vi "calculateRoll.vi"(9 "az":dbl, 10 "ay":dbl) -> (3 "roll":dbl)   [LabVIEW 2019]
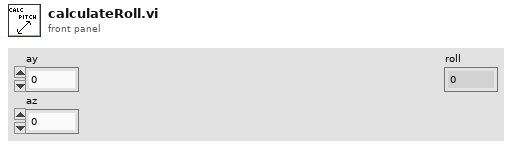
[diagram p1: front panel]
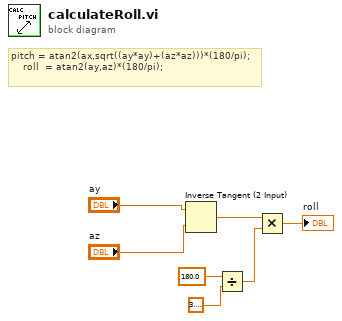
[diagram p0: block diagram]
diagram:
  # "pitch = atan2(ax,sqrt((ay*ay)+(az*az)))*(180/pi);\n    roll  = atan2(ay,az)*(180/pi);"
  n1 = Inverse Tangent (2 Input)(1:"az", 2:"ay") -> (0:w7:dbl)
  n2 = Divide(x=180.0, y=3.141592653589793) -> (x/y=w4:dbl)
  n3 = Multiply(x=w7, y=w4) -> (x*y=→"roll":dbl)
